vi "WD Polling.vi"() -> ()   [LabVIEW 2015]
doc: "This VI will set an indicator to true if the whack control is not set prior to the expiration of each timeout (in ms). The Arm control is set to SWITCH1 and the Whack control is set to PB1."
uses:
  <vilib>/rvi/Emulation/niFpgaGetClockAttributes.vi
  <vilib>/rvi/Emulation/niFpgaSctlEmulationGetInTimedLoop.vi
  <vilib>/rvi/Emulation/niFpgaEmulationReportErrorSimple.vi
  Instance           1 20Saved   WD - Polling .vi
  <vilib>/rvi/eio/common/nirviEmuTemplateMethod_errors.vi
  <vilib>/rvi/Emulation/niFpgaCriticalErrorInLSC.vi
  <vilib>/eio/EIONode/EIONode.xnode
panel:
  in  "Arm":bool
  in  "Whack":bool
  in  "Timeout (ms)":u32=500
  out "Expired":bool
  # "This VI sets the Expired indicator and LED 1 to true if the whack \ncontrol is not set prior to the expiration of each timeout (in ms). \nThe Arm and Whack controls are set on the RT Watchdog Occurance \nVI front panel instead of PB1 and PB2 as in the previous example,\n and passed to the FPGA VI via Read/Write Controls."
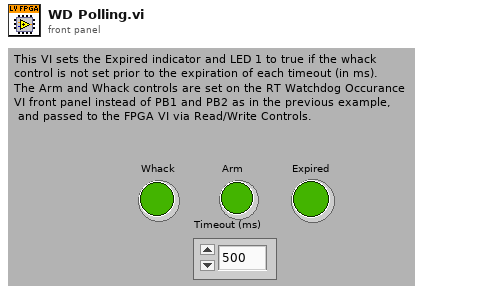
[diagram p1: front panel]
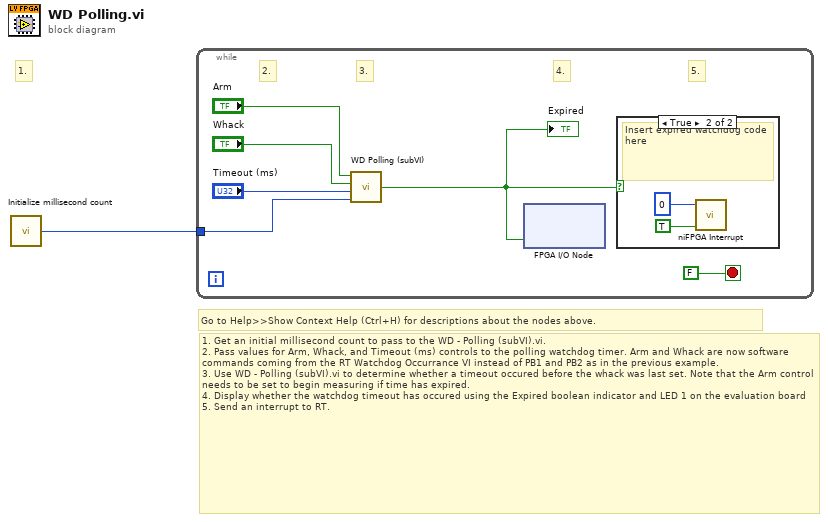
[diagram p0: block diagram]
diagram:
  # "Go to Help>>Show Context Help (Ctrl+H) for descriptions about the nodes above."
  # "1."
  # "1. Get an initial millisecond count to pass to the WD - Polling (subVI).vi.\n2. Pass values for Arm, Whack, and Timeout (ms) controls to the polling watchdog timer. Arm and Whack are now software commands coming from the RT Watchdog Occurrance VI instead of PB1 and PB2 as in the previous example.\n3. Use WD - Polling (subVI).vi to determine whether a timeout occured before the whack was last set. Note that the Arm control needs to be set to begin measuring if time has expired.\n4. Display whether the watchdog timeout has occured using the Expired boolean indicator and LED 1 on the evaluation board\n5. Send an interrupt to RT."
  n1 = call "Initialize millisecond count"() -> ("Tick Count(mSec)"=w1:u32)
  n2 = while {
    tunnel: w1 -> [w7]
    stop <- FALSE stop-if-true
    # "4."
    # "5."
    # "3."
    # "2."
    n3 = call "WD Polling (subVI).vi"("Timer Initialize (ms)"=w7, "Timeout (ms)"="Timeout (ms)", "Whack"="Whack", "Arm"="Arm") -> ("Expired"=w2:bool)  [unwired: 2 out]
    "Expired" <- w2
    n4 = xnode "FPGA I/O Node"("LED 1"=w2) -> ()  [unwired: 1 in, 1 out]
    n5 = case shown="True" w2 {
      frame False {
      }
      frame True {
        # "Insert expired watchdog code here"
        n6 = call <vilib>:"niFPGA Interrupt.vi"("Wait Until Cleared (F)"=TRUE ("Wait Until Cleared"), "IRQ Number (0)"=u8 0 ("IRQ Bit (0-31)")) -> ()  [unwired: 1 in]
      }
    }
  }
